vi "configure.vi"(8 "error in (no error)":errorcluster, 11 "DL090215DataCollection in":refnum<class "DataCollectionDL090215.lvclass">) -> (0 "error out":errorcluster, 3 "DL090215DataCollection out":refnum<class "DataCollectionDL090215.lvclass">)   [LabVIEW 2010, in "DataCollectionDL090215.lvclass"]
uses:
  DataCollectionDL090215.lvclass
  DataCollectionDL090215.lvclass/DataCollectionDL090215.ctl
  common/classes/Image/Image/target_format_enum.ctl
  common/classes/ErrorController/ErrorController/class_data.vi
  common/classes/GenericComponent/GenericComponent/GenericComponent.lvclass
  common/classes/ErrorController/ErrorController/ErrorController.lvclass
panel:
  in  "writing OME header as default?":bool=TRUE
  in  "format":T1(ring)
  in  "autosave as default?":bool=TRUE
  out "configuration":string
  in  "cancel":bool
  in  "save":bool
  in  "channels in same file":bool
  # "Configure DataCollectionDL090215"
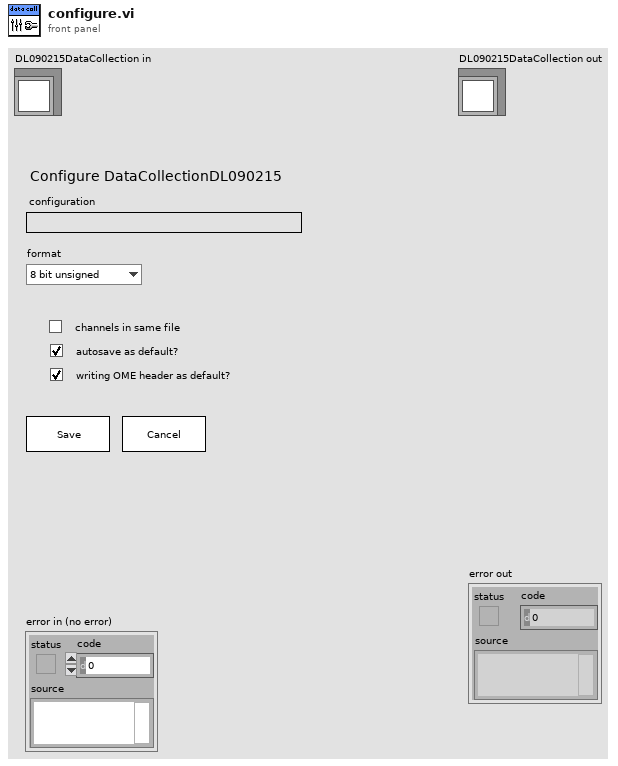
[diagram p1: front panel]
types:
  T1 = enum16{"8 bit unsigned", "16 bit unsigned", "16 bit signed", "32 bit unsigned", "32 bit signed"}
  T2 = typedef "target_format_enum.ctl" = enum16{"don't force", "uint8", "uint16", "int16", "uint32", "int32", "single float"}
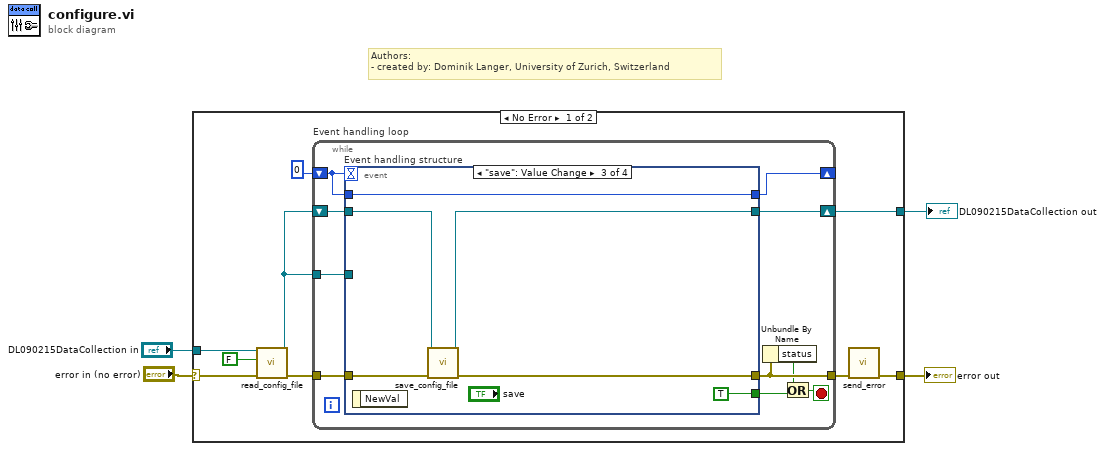
[diagram p0: block diagram]
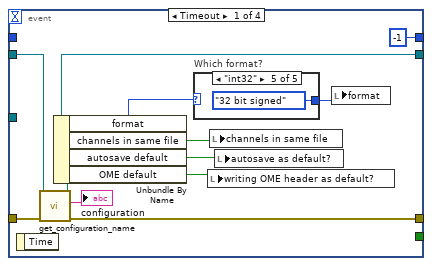
[diagram p2: hidden frame]
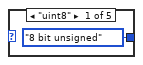
[diagram p3: hidden frame]
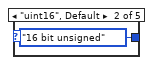
[diagram p4: hidden frame]
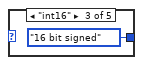
[diagram p5: hidden frame]
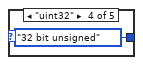
[diagram p6: hidden frame]
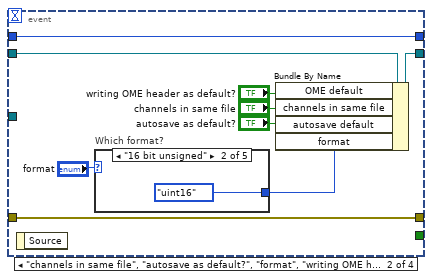
[diagram p7: hidden frame]
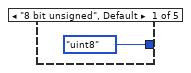
[diagram p8: hidden frame]
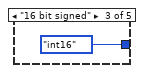
[diagram p9: hidden frame]
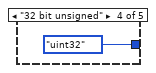
[diagram p10: hidden frame]
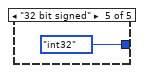
[diagram p11: hidden frame]
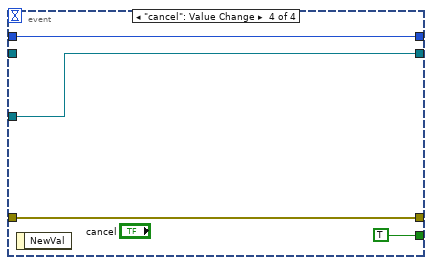
[diagram p12: hidden frame]
diagram:
  # "Authors: \n- created by: Dominik Langer, University of Zurich, Switzerland"
  n1 = case shown="No Error" "error in (no error)" {
    selector: "error in (no error)" -> [w11 w65]
    tunnel: [w7 w65] -> w3
    tunnel: [w12 w64] -> w1
    tunnel: "DL090215DataCollection in" -> [w9 w64]
    frame No Error {
      n2 = call-dynamic "read_config_file.vi"("error in (no error)"=w11, "force load?"=FALSE, "GenericPlugin in"=w9) -> ("error out"=w10:errorcluster, "GenericPlugin out"=w5:refnum<class "DataCollectionDL090215.lvclass">)  [unwired: 7 out]
      n3 = while "Event handling loop" {
        shift-right: [w21] -> _
        shift-left: 0 -> [w22]
        shift-right: [w19] -> w12
        shift-left: w5 -> [w20]
        tunnel: w10 -> [w23]
        tunnel: [w18] -> w6
        tunnel: w5 -> [w14]
        stop <- w15 stop-if-true
        n4 = event "Event handling structure" shown="[2] \"save\": Value Change" {
          selector: _ -> [_ _ _ _]
          dyn-events: _ -> [_ _ _ _]
          timeout: w22 -> [_ _ _ _]
          tunnel: w23 -> [w32 w47 w57 w61]
          tunnel: [-1 w48 w59 w63] -> w21
          tunnel: w22 -> [_ w48 w59 w63]
          tunnel: [_ _ TRUE TRUE] -> w17
          tunnel: [w25 w47 w56 w61] -> w18
          tunnel: w20 -> [w31 w46 w54 _]
          tunnel: [w30 w45 w55 w60] -> w19
          tunnel: w14 -> [_ _ _ w60]
          event Timeout {
            n5 = event-data() -> ()  [unwired: 2 out]
            n6 = call "get_configuration_name.vi"("error in (no error)"=w32, "GenericPlugin.lvclass in"=w31) -> ("error out"=w25:errorcluster, "configuration name"=→"configuration":string, "GenericPlugin.lvclass out"=w30:refnum<class "DataCollectionDL090215.lvclass">)  [unwired: 7 in]
            n7 = Unbundle By Name(w30) -> ("format"=w27:T2, "channels in same file"=w33:bool, "autosave default"=w28:bool, "OME default"=w24:bool)
            n8 = case "Which format?" shown="\"int32\"" w27 {
              tunnel: [T1."8 bit unsigned" ("format") T1."16 bit unsigned" ("format") T1."16 bit signed" ("format") T1."32 bit unsigned" ("format") T1."32 bit signed" ("format")] -> w26
              frame "uint8" {
              }
              frame "uint16", Default {
              }
              frame "int16" {
              }
              frame "uint32" {
              }
              frame "int32" {
              }
            }
            n9 = local write "writing OME header as default?"(w24) -> ()
            n10 = local write "channels in same file"(w33) -> ()
            n11 = local write "autosave as default?"(w28) -> ()
            n12 = local write "format"(w26) -> ()
          }
          event "channels in same file", "autosave as default?", "format", "writing OME header as default?": Value Change {
            n13 = event-data() -> ()  [unwired: 2 out]
            n14 = case "Which format?" shown="\"16 bit unsigned\"" "format" {
              tunnel: [target_format_enum."uint8" ("configuration data.saving format.format") target_format_enum."uint16" ("configuration data.saving format.format") target_format_enum."int16" ("configuration data.saving format.format") target_format_enum."uint32" ("configuration data.saving format.format") target_format_enum."int32" ("configuration data.saving format.format")] -> w41
              frame "8 bit unsigned", Default {
              }
              frame "16 bit unsigned" {
              }
              frame "16 bit signed" {
              }
              frame "32 bit unsigned" {
              }
              frame "32 bit signed" {
              }
            }
            n15 = Bundle By Name(cluster=w46, "OME default"="writing OME header as default?", "channels in same file"="channels in same file", "autosave default"="autosave as default?", "format"=w41) -> (w45:refnum<class "DataCollectionDL090215.lvclass">)
          }
          event "save": Value Change {
            n16 = event-data() -> ()  [unwired: 2 out]
            n17 = call-dynamic "save_config_file.vi"("error in (no error)"=w57, "GenericPlugin in"=w54) -> ("error out"=w56:errorcluster, "GenericPlugin out"=w55:refnum<class "DataCollectionDL090215.lvclass">)  [unwired: 2 in, 6 out]
          }
          event "cancel": Value Change {
            n18 = event-data() -> ()  [unwired: 2 out]
          }
        }
        n19 = Unbundle By Name(w18) -> ("status"=w16:bool)
        n20 = Or(x=w16, y=w17) -> (x .or. y?=w15:bool)
      }
      n21 = call "send_error.vi"("error in (no error)"=w6) -> ("error out"=w7:errorcluster)  [unwired: 10 in]
    }
    frame Error {
    }
  }
  "error out" <- w3
  "DL090215DataCollection out" <- w1
